vi "zadanie_1.vi"() -> ()   [LabVIEW 2020]
panel:
  out "String":string
  out "x2":dbl
  out "x1":dbl
  in  "c":dbl
  in  "b":dbl
  in  "a":dbl
  # "x^2+"
  # "x+"
  # "=0"
  # "Ma nastepujace pierwiastki"
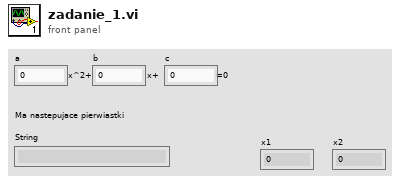
[diagram p1: front panel]
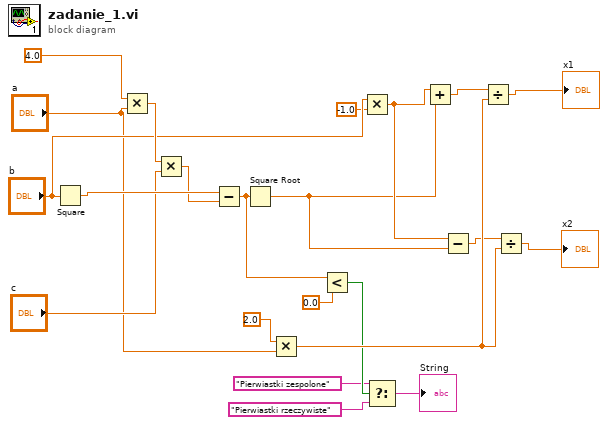
[diagram p0: block diagram]
diagram:
  n1 = Square(x="b") -> (x^2=w22:dbl)
  n2 = Multiply(x=4.0, y="a") -> (x*y=w20:dbl)
  n3 = Multiply(x=w20, y="c") -> (x*y=w18:dbl)
  n4 = Subtract(x=w22, y=w18) -> (x-y=w1:dbl)
  n5 = Square Root(x=w1) -> (sqrt(x)=w7:dbl)
  n6 = Multiply(x=2.0, y="a") -> (x*y=w12:dbl)
  n7 = Less?(x=w1, y=0.0) -> (x < y?=w5:bool)
  n8 = Multiply(x="b", y=-1.0) -> (x*y=w15:dbl)
  n9 = Select(t="Pierwiastki zespolone", s=w5, f="Pierwiastki rzeczywiste") -> (s? t:f=→"String":string)
  n10 = Add(x=w15, y=w7) -> (x+y=w11:dbl)
  n11 = Subtract(x=w15, y=w7) -> (x-y=w10:dbl)
  n12 = Divide(x=w11, y=w12) -> (x/y=→"x1":dbl)
  n13 = Divide(x=w10, y=w12) -> (x/y=→"x2":dbl)
